vi "FPGA EXPANSION 9149.vi"() -> ()   [LabVIEW 2018]
uses:
  controls/Pipeline T&P.ctl
  controls/In Tank T&P.ctl
  <vilib>/Platform/TimedLoop/XDataNode/timing_clust.ctl
  <vilib>/Platform/TimedLoop/XDataNode/nitl_modes.ctl
  <vilib>/Platform/TimedLoop/XDataNode/wakeup.ctl
  <vilib>/rvi/FXPMathLib/basic elements/FxpIntAccumulator/subVIs/nifxpmath_IntAccumulator_SimConfig.ctl
  <vilib>/rvi/Emulation/niFpgaGetClockAttributes.vi
  <vilib>/rvi/Emulation/niFpgaSctlEmulationGetInTimedLoop.vi
  <vilib>/rvi/Emulation/niFpgaEmulationReportErrorSimple.vi
  <vilib>/rvi/eio/common/nirviEmuTemplateMethod_errors.vi
  <vilib>/rvi/Analysis/common/codeGenErrors/XNode/niFpgaXNodeCodeGenErrorHandle.vi
  <vilib>/rvi/Emulation/niFpgaCriticalErrorInLSC.vi
  <vilib>/rvi/FXPMathLib/basic elements/FxpIntAccumulator/simVIs/DllFxpIntAccumulator_sub.vi
  <vilib>/rvi/Emulation/niFpgaProcessEmulError.vi
  <vilib>/eio/EIONode/EIONode.xnode
  <vilib>/rvi/Analysis/measure/mean-var-std/XNode/niFpgaMean-Var-Std.xnode
  <vilib>/Platform/TimedLoop/XDataNode/XDataNode.xnode
  <vilib>/rvi/FXPMathLib/basic elements/FxpIntAccumulator/XNode/nifxpmath_IntAccumulator.xnode
  <vilib>/rvi/FXPMathLib/FxpMul/XNode/nifxpmath_Multiplier.xnode
  <vilib>/Platform/TimedLoop/XDataNode/XDNodeRunTimeDep.lvlib
  <vilib>/rvi/FXPMathLib/sim/FxpSim.dll
panel:
  out "error out":errorcluster
  out "In Tank T&P":T1 {"LOX Tank Temp.[F]" scale=0.0..100.0; "LOX Tank Press. [psi]" scale=0.0..10.0; "LNG Tank Temp. [F]" scale=0.0..100.0; "LNG Tank Press. [psi]" scale=0.0..10.0}
  out "Pipeline T&P":T2 {"LOX UST" scale=0.0..100.0; "LOX MST" scale=0.0..100.0; "LOX DST" scale=0.0..100.0; "LNG UST" scale=0.0..100.0; "LNG MST" scale=0.0..100.0; "LNG DST" scale=0.0..100.0; "LOX USP" scale=0.0..10.0; "LOX MSP" scale=0.0..10.0; "LOX DST" scale=0.0..10.0; "LNG USP" scale=0.0..10.0; "LNG MSP" scale=0.0..10.0; "LNG DSP" scale=0.0..10.0}
  out "Tick Count(mSec)":u32
  in  "Enable Watchdog":bool
  in  "Pet Watchdog":bool
  in  "Watchdog Timeout Period (ticks)":u64=40000000 format="%.0p"
  out "Watchdog Timed Out?":bool=TRUE
  out "Time Since Last Pet":u64
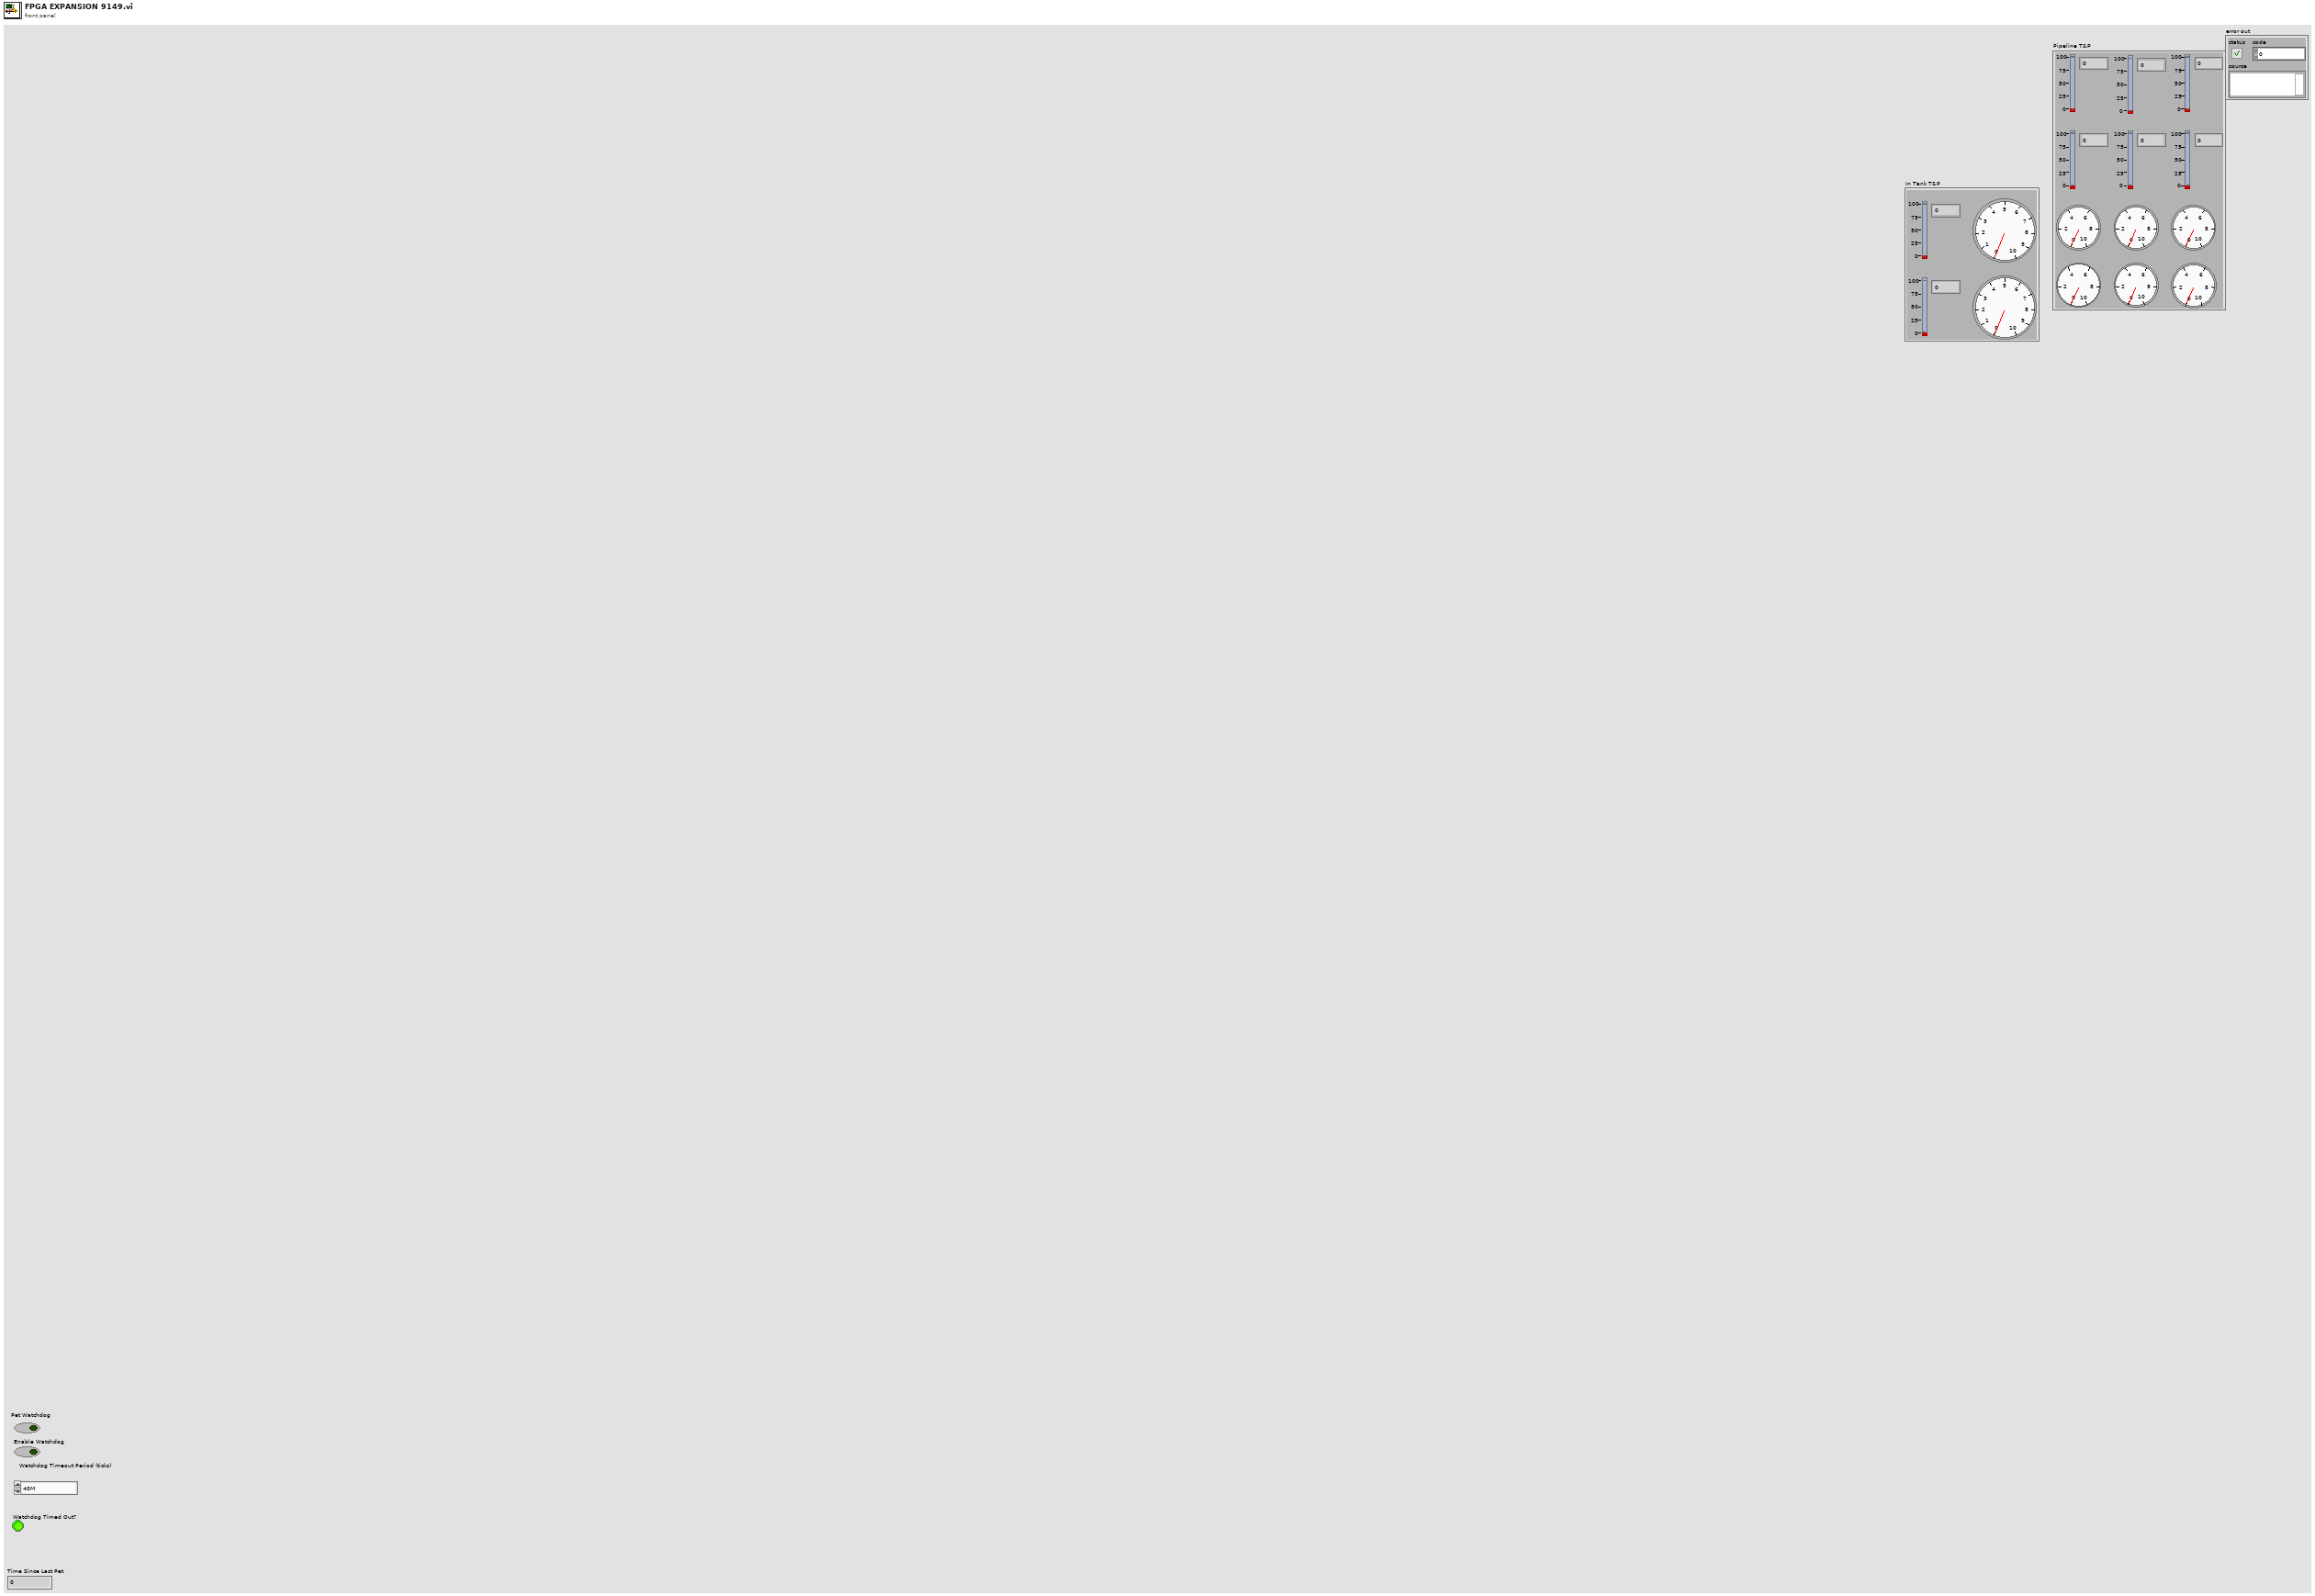
[diagram p1: front panel]
types:
  T1 = typedef "In Tank T&P.ctl" = cluster{"LOX Tank Temp.[F]":sgl, "LOX Tank Press. [psi]":sgl, "LNG Tank Temp. [F]":sgl, "LNG Tank Press. [psi]":sgl}
  T2 = typedef "Pipeline T&P.ctl" = cluster{"LOX UST":sgl, "LOX MST":sgl, "LOX DST":sgl, "LNG UST":sgl, "LNG MST":sgl, "LNG DST":sgl, "LOX USP":sgl, "LOX MSP":sgl, "LOX DST":sgl, "LNG USP":sgl, "LNG MSP":sgl, "LNG DSP":sgl}
  T3 = typedef "XDNodeRunTimeDep.lvlib/timing_clust.ctl" = cluster{"Expected End [f-1]":u64, "Actual End [f-1]":u64, "Finished Late? [f-1]":bool, "Expected End [i-1]":u64, "Actual End [i-1]":u64, "Finished Late? [i-1]":bool, "Expected Start [i]":u64, "Actual Start [i]":u64, "Expected Start [f]":u64, "Actual Start [f]":u64, "Source Name":string, "Structure Name":string, "Period":i64, "Deadline":i64, "Offset":i64, "Start":i64, "Priority":i32, "Timeout":i32, "Mode":T4, "Wakeup Reason":T5, "Error":errorcluster, "Source Type":string, "Secondary Source Type":string, "Global End Time":u64, "Global Start Time":u64, "Frame Duration":u64, "Iteration Duration":u64, "Assigned CPU":i32, "I/O Scan Engine Mode":u32}
  T4 = typedef "XDNodeRunTimeDep.lvlib/nitl_modes.ctl" = enum32{"No Change", "Process missed periods, maintain original phase", "Discard missed periods, maintain original phase", "Process missed periods, ignore original phase", "Discard missed periods, ignore original phase"}
  T5 = typedef "XDNodeRunTimeDep.lvlib/wakeup.ctl" = enum32{"Normal", "Aborted", "Asynchronous wakeup", "Timing source error", "Timed loop error", "Timeout"}
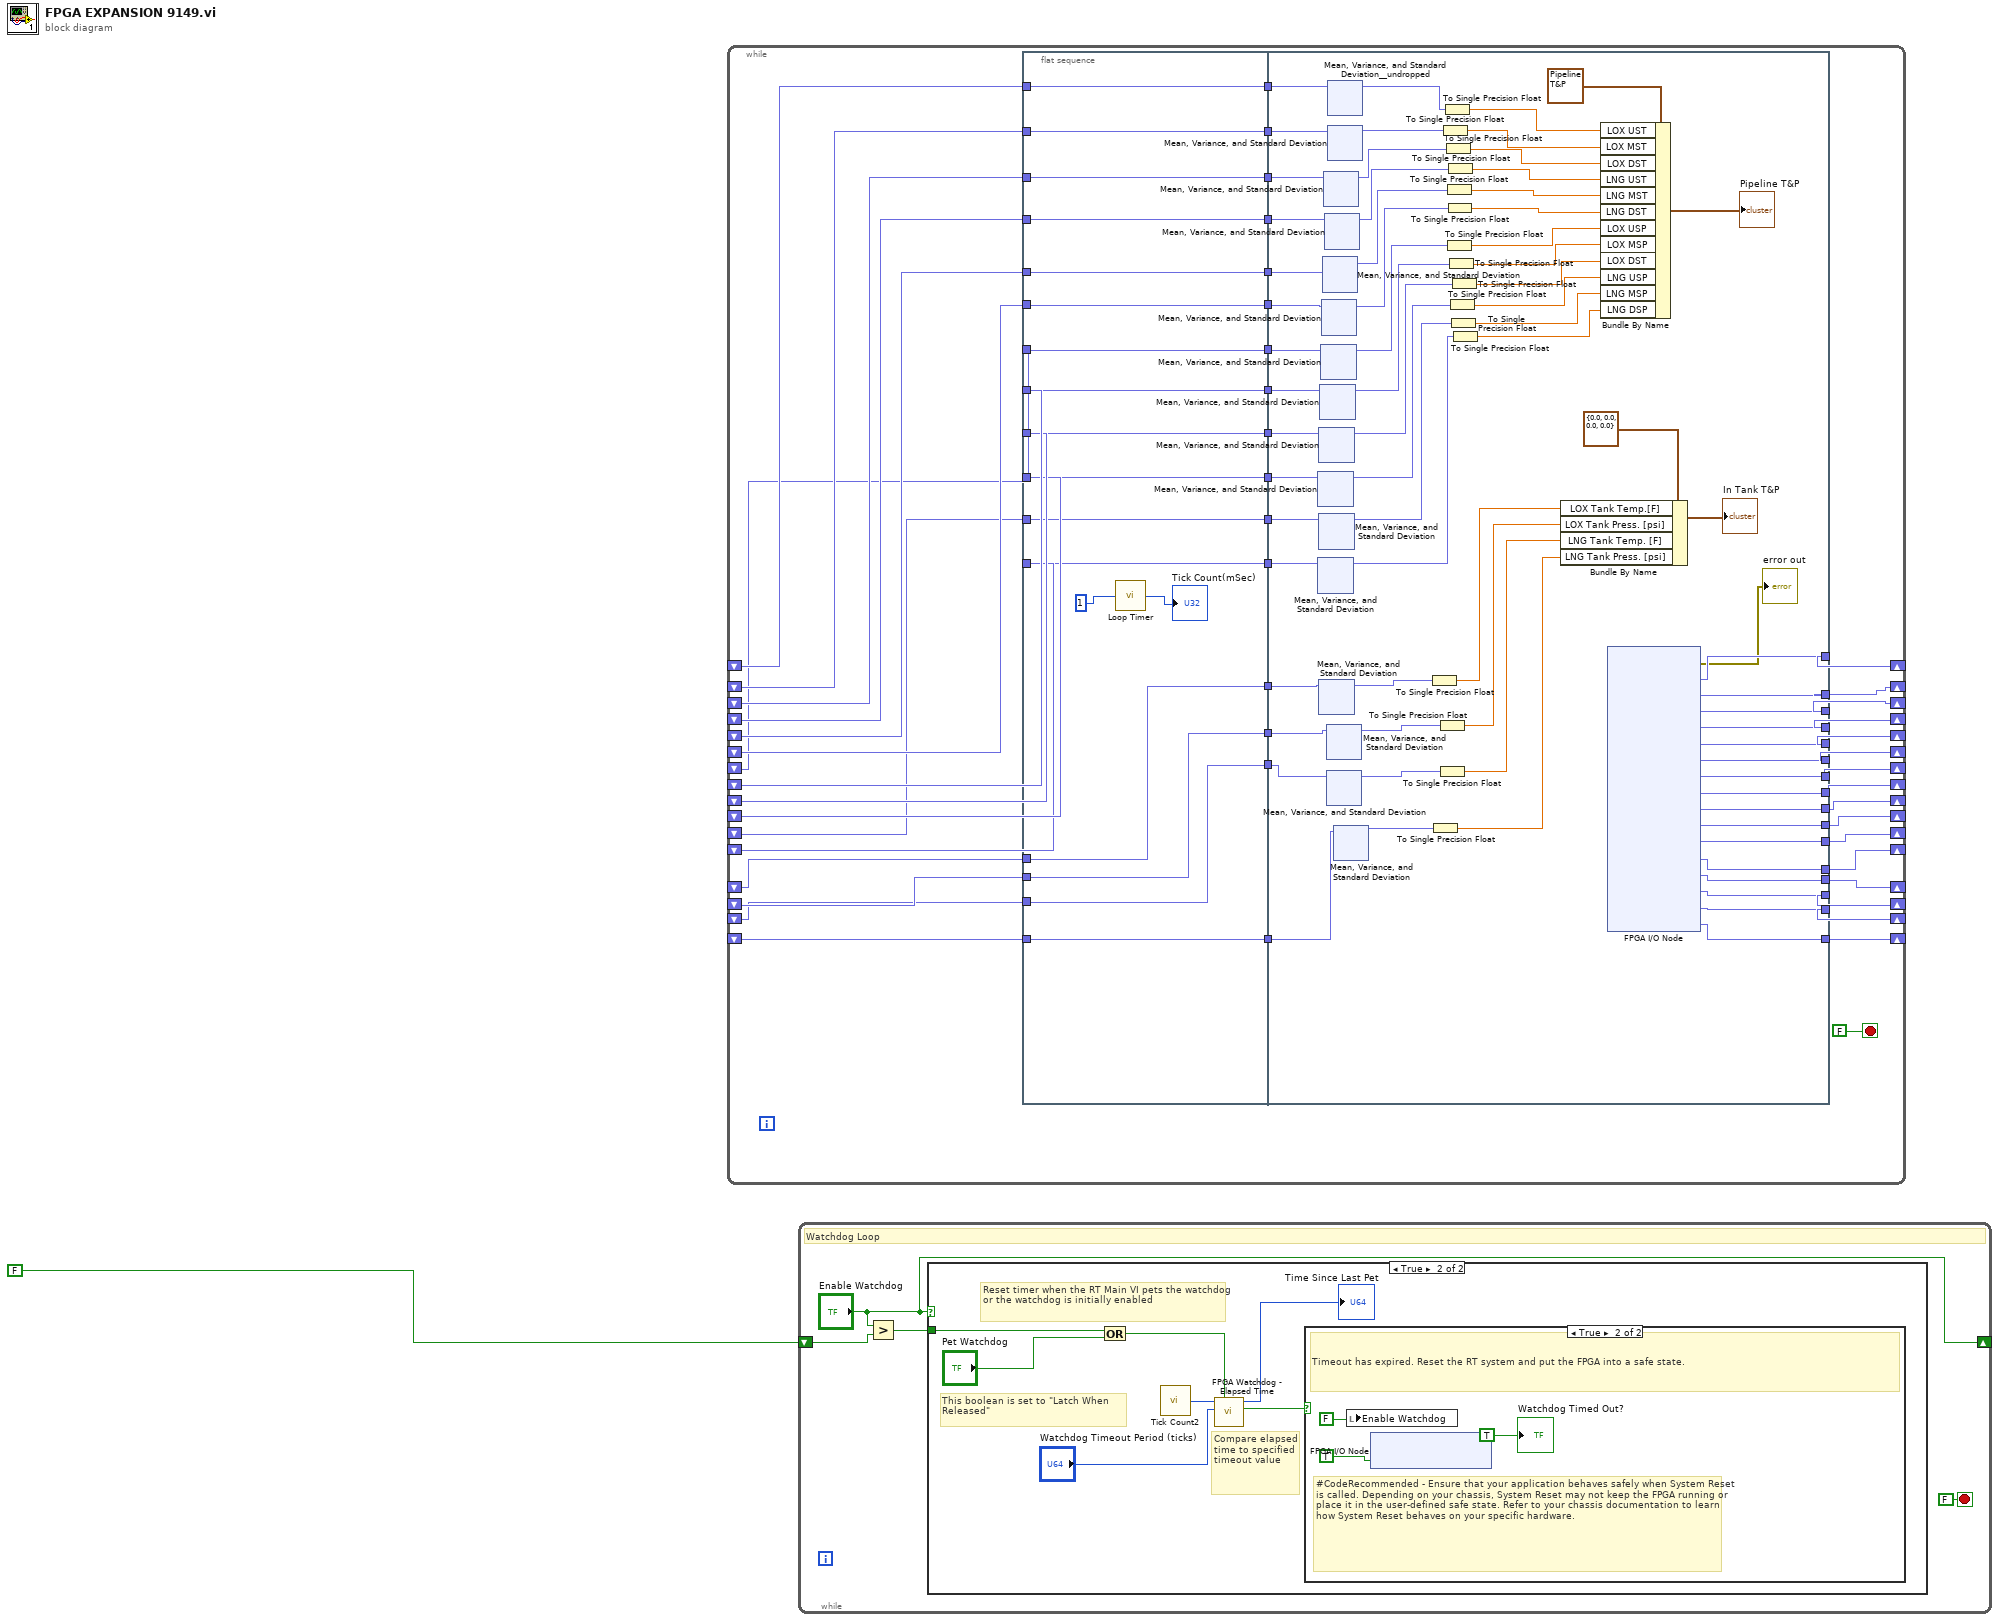
[diagram p0: block diagram]
diagram:
  n1 = while {
    shift-right: [w38] -> _
    shift-left: _ -> [w27]
    shift-right: [w39] -> _
    shift-left: _ -> [w14]
    shift-right: [w40] -> _
    shift-left: _ -> [w28]
    shift-right: [w41] -> _
    shift-left: _ -> [w29]
    shift-right: [w42] -> _
    shift-left: _ -> [w30]
    shift-right: [w43] -> _
    shift-left: _ -> [w31]
    shift-right: [w44] -> _
    shift-left: _ -> [w32]
    shift-right: [w45] -> _
    shift-left: _ -> [w33]
    shift-right: [w46] -> _
    shift-left: _ -> [w35]
    shift-right: [w47] -> _
    shift-left: _ -> [w36]
    shift-right: [w48] -> _
    shift-left: _ -> [w34]
    shift-right: [w49] -> _
    shift-left: _ -> [w37]
    shift-right: [w13] -> _
    shift-left: _ -> [w10]
    shift-right: [w12] -> _
    shift-left: _ -> [w9]
    shift-right: [w11] -> _
    shift-left: _ -> [w8]
    shift-right: [w4] -> _
    shift-left: _ -> [w3]
    stop <- FALSE stop-if-true
    n2 = flat-sequence {
      tunnel: w27 -> [w57]
      tunnel: w14 -> [w58]
      tunnel: w28 -> [w59]
      tunnel: w29 -> [w60]
      tunnel: w30 -> [w61]
      tunnel: w31 -> [w62]
      tunnel: w32 -> [w63]
      tunnel: w33 -> [w64]
      tunnel: w34 -> [w65]
      tunnel: w35 -> [w66]
      tunnel: w36 -> [w67]
      tunnel: w37 -> [w68]
      tunnel: [w68] -> w26
      tunnel: [w67] -> w25
      tunnel: [w66] -> w24
      tunnel: [w65] -> w23
      tunnel: [w64] -> w22
      tunnel: [w63] -> w21
      tunnel: [w62] -> w20
      tunnel: [w61] -> w19
      tunnel: [w60] -> w18
      tunnel: [w59] -> w17
      tunnel: [w58] -> w16
      tunnel: [w57] -> w15
      tunnel: w10 -> [w54]
      tunnel: w9 -> [w53]
      tunnel: w8 -> [w52]
      tunnel: [w54] -> w7
      tunnel: [w53] -> w6
      tunnel: [w52] -> w5
      tunnel: w3 -> [w51]
      tunnel: [w51] -> w2
      tunnel: [w137] -> w49
      tunnel: [w136] -> w48
      tunnel: [w135] -> w47
      tunnel: [w134] -> w46
      tunnel: [w133] -> w45
      tunnel: [w132] -> w44
      tunnel: [w131] -> w43
      tunnel: [w130] -> w42
      tunnel: [w129] -> w41
      tunnel: [w128] -> w40
      tunnel: [w127] -> w39
      tunnel: [w126] -> w38
      tunnel: w26 -> [w125]
      tunnel: w25 -> [w124]
      tunnel: w24 -> [w123]
      tunnel: w23 -> [w122]
      tunnel: w22 -> [w121]
      tunnel: w21 -> [w120]
      tunnel: w20 -> [w119]
      tunnel: w19 -> [w118]
      tunnel: w18 -> [w117]
      tunnel: w17 -> [w116]
      tunnel: w16 -> [w115]
      tunnel: w15 -> [w114]
      tunnel: [w88] -> w13
      tunnel: [w87] -> w12
      tunnel: [w86] -> w11
      tunnel: w7 -> [w85]
      tunnel: w6 -> [w84]
      tunnel: w5 -> [w83]
      tunnel: [w73] -> w4
      tunnel: w2 -> [w70]
      frame #0 {
        n3 = call "Loop Timer"("Count(uSec)"=u32 1 ("Count(mSec)")) -> ("Tick Count(uSec)"=→"Tick Count(mSec)":u32)
      }
      frame #1 {
        n4 = xnode "Mean, Variance, and Standard Deviation"("input data"=w116) -> ("mean"=w104:fxp<+/-,24,5>)  [unwired: 1 in, 1 out]
        n5 = xnode "Mean, Variance, and Standard Deviation"("input data"=w114) -> ("mean"=w102:fxp<+/-,24,5>)  [unwired: 1 in, 1 out]
        n6 = xnode "Mean, Variance, and Standard Deviation"("input data"=w117) -> ("mean"=w105:fxp<+/-,24,5>)  [unwired: 1 in, 1 out]
        n7 = xnode "Mean, Variance, and Standard Deviation"("input data"=w115) -> ("mean"=w103:fxp<+/-,24,5>)  [unwired: 1 in, 1 out]
        n8 = xnode "Mean, Variance, and Standard Deviation"("input data"=w85) -> ("mean"=w80:fxp<+/-,24,5>)  [unwired: 1 in, 1 out]
        n9 = xnode "Mean, Variance, and Standard Deviation"("input data"=w118) -> ("mean"=w106:fxp<+/-,24,5>)  [unwired: 1 in, 1 out]
        n10 = xnode "Mean, Variance, and Standard Deviation"("input data"=w119) -> ("mean"=w107:fxp<+/-,24,5>)  [unwired: 1 in, 1 out]
        n11 = xnode "Mean, Variance, and Standard Deviation"("input data"=w120) -> ("mean"=w108:fxp<+/-,24,5>)  [unwired: 1 in, 1 out]
        n12 = xnode "Mean, Variance, and Standard Deviation"("input data"=w121) -> ("mean"=w109:fxp<+/-,24,5>)  [unwired: 1 in, 1 out]
        n13 = xnode "Mean, Variance, and Standard Deviation"("input data"=w124) -> ("mean"=w111:fxp<+/-,24,5>)  [unwired: 1 in, 1 out]
        n14 = xnode "Mean, Variance, and Standard Deviation"("input data"=w123) -> ("mean"=w110:fxp<+/-,24,5>)  [unwired: 1 in, 1 out]
        n15 = xnode "Mean, Variance, and Standard Deviation"("input data"=w84) -> ("mean"=w81:fxp<+/-,24,5>)  [unwired: 1 in, 1 out]
        n16 = xnode "Mean, Variance, and Standard Deviation"("input data"=w83) -> ("mean"=w82:fxp<+/-,24,5>)  [unwired: 1 in, 1 out]
        n17 = xnode "Mean, Variance, and Standard Deviation__undropped"("input data"=w125) -> ("mean"=w113:fxp<+/-,24,5>)  [unwired: 1 in, 1 out]
        n18 = xnode "Mean, Variance, and Standard Deviation"("input data"=w122) -> ("mean"=w112:fxp<+/-,24,5>)  [unwired: 1 in, 1 out]
        n19 = xnode "Mean, Variance, and Standard Deviation"("input data"=w70) -> ("mean"=w72:fxp<+/-,24,5>)  [unwired: 1 in, 1 out]
        n20 = To Single Precision Float(number=w80) -> (single precision float=w76:sgl)
        n21 = To Single Precision Float(number=w72) -> (single precision float=w71:sgl)
        n22 = To Single Precision Float(number=w81) -> (single precision float=w75:sgl)
        n23 = To Single Precision Float(number=w82) -> (single precision float=w74:sgl)
        n24 = To Single Precision Float(number=w112) -> (single precision float=w100:sgl)
        n25 = To Single Precision Float(number=w113) -> (single precision float=w101:sgl)
        n26 = To Single Precision Float(number=w111) -> (single precision float=w99:sgl)
        n27 = To Single Precision Float(number=w109) -> (single precision float=w97:sgl)
        n28 = To Single Precision Float(number=w107) -> (single precision float=w95:sgl)
        n29 = To Single Precision Float(number=w108) -> (single precision float=w96:sgl)
        n30 = To Single Precision Float(number=w110) -> (single precision float=w98:sgl)
        n31 = To Single Precision Float(number=w106) -> (single precision float=w94:sgl)
        n32 = To Single Precision Float(number=w104) -> (single precision float=w92:sgl)
        n33 = To Single Precision Float(number=w103) -> (single precision float=w91:sgl)
        n34 = To Single Precision Float(number=w105) -> (single precision float=w93:sgl)
        n35 = To Single Precision Float(number=w102) -> (single precision float=w77:sgl)
        n36 = Bundle By Name(cluster=T1 {"LOX Tank Temp.[F]"=0.0, "LOX Tank Press. [psi]"=0.0, "LNG Tank Temp. [F]"=0.0, "LNG Tank Press. [psi]"=0.0} ("output cluster 3"), "LOX Tank Temp.[F]"=w76, "LOX Tank Press. [psi]"=w75, "LNG Tank Temp. [F]"=w74, "LNG Tank Press. [psi]"=w71) -> (→"In Tank T&P":T1)
        n37 = Bundle By Name(cluster=T2 {"LOX UST"=0.0, "LOX MST"=0.0, "LOX DST"=0.0, "LNG UST"=0.0, "LNG MST"=0.0, "LNG DST"=0.0, "LOX USP"=0.0, "LOX MSP"=0.0, "LOX DST"=0.0, "LNG USP"=0.0, "LNG MSP"=0.0, "LNG DSP"=0.0} ("output cluster 2"), "LOX UST"=w101, "LOX MST"=w100, "LOX DST"=w99, "LNG UST"=w98, "LNG MST"=w97, "LNG DST"=w96, "LOX USP"=w95, "LOX MSP"=w94, "LOX DST"=w93, "LNG USP"=w92, "LNG MSP"=w91, "LNG DSP"=w77) -> (→"Pipeline T&P":T2)
        n38 = xnode "FPGA I/O Node"() -> ("error out"=→"error out":errorcluster, "Mod1/AI0"=w137:fxp<+/-,24,5>, "Mod1/AI1"=w136:fxp<+/-,24,5>, "Mod1/AI2"=w135:fxp<+/-,24,5>, "Mod1/AI3"=w134:fxp<+/-,24,5>, "Mod2/AI0"=w133:fxp<+/-,24,5>, "Mod2/AI1"=w132:fxp<+/-,24,5>, "Mod2/AI2"=w131:fxp<+/-,24,5>, "Mod2/AI3"=w130:fxp<+/-,24,5>, "Mod3/AI0"=w129:fxp<+/-,24,5>, "Mod3/AI1"=w128:fxp<+/-,24,5>, "Mod3/AI2"=w127:fxp<+/-,24,5>, "Mod3/AI3"=w126:fxp<+/-,24,5>, "Mod4/AI0"=w88:fxp<+/-,24,5>, "Mod4/AI1"=w87:fxp<+/-,24,5>, "Mod4/AI2"=w86:fxp<+/-,24,5>, "Mod4/AI3"=w73:fxp<+/-,24,5>)  [unwired: 17 in, 16 out]
      }
    }
  }
  n39 = while "RT Watchdog Loop" {
    shift-right: ["Enable Watchdog"] -> _
    shift-left: FALSE ("Enable RT Watchdog") -> [w1357]
    stop <- FALSE stop-if-true
    # "Watchdog Loop"
    n40 = Greater?(x="Enable Watchdog", y=w1357) -> (0:w1354:bool)
    n41 = case shown="True" "Enable Watchdog" {
      tunnel: w1354 -> [_ w1360]
      frame False {
        # "This loop has to be explicitly enabled from the RT Main VI.  This reduces the possiblity of an endless reboot cycle."
      }
      frame True {
        # "This boolean is set to \"Latch When Released\""
        # "Compare elapsed time to specified timeout value"
        # "Reset timer when the RT Main VI pets the watchdog or the watchdog is initially enabled"
        n42 = Or(x=w1360, y="Pet Watchdog") -> (x .or. y?=w1359:bool)
        n43 = call "Tick Count2"() -> ("Tick Count(Ticks)"=w1363:u32)
        n44 = call "FPGA Watchdog - Elapsed Time.vi"("Reset"=w1359, "Timeout Period"="Watchdog Timeout Period (ticks)", "Current Time"=w1363) -> ("Timeout"=w1358:bool, "Elapsed Time"=→"Time Since Last Pet":u64)  [unwired: 7 in]
        n45 = case shown="True" w1358 {
          frame False {
            # "Timeout has not expired."
          }
          frame True {
            # "#CodeRecommended - Ensure that your application behaves safely when System Reset is called. Depending on your chassis, System Reset may not keep the FPGA running or place it in the user-defined safe state. Refer to your chassis documentation to learn how System Reset behaves on your specific hardware."
            # "Timeout has expired. Reset the RT system and put the FPGA into a safe state."
            n46 = local write "Enable Watchdog"(FALSE ("Enable RT Watchdog")) -> ()
            n47 = xnode "FPGA I/O Node"("USER FPGA LED"=TRUE ("RT Reset on Watchdog Failure?")) -> ()  [unwired: 1 in, 1 out]
            "Watchdog Timed Out?" <- TRUE ("Watchdog Timed Out?")
          }
        }
      }
    }
  }
